vi "Variable_Local.vi"() -> ()   [LabVIEW 2016]
panel:
  out "String 2":string
  in  "String":string
  out "Waveform Chart":dbl(graph)
  in  "Stop Button":bool
  out "Numeric Control 2":i32
  out "Numeric Control":i32
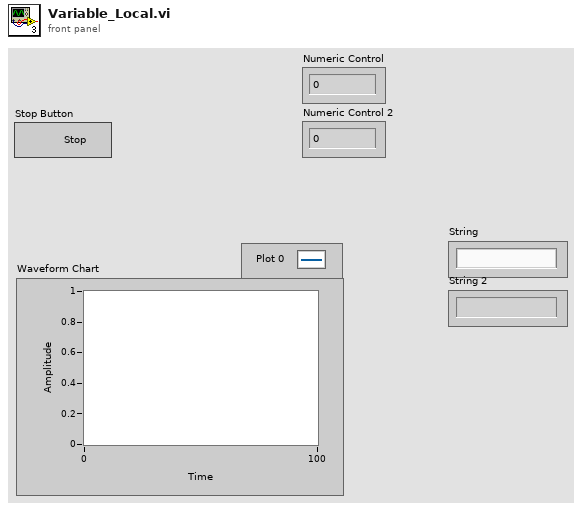
[diagram p1: front panel]
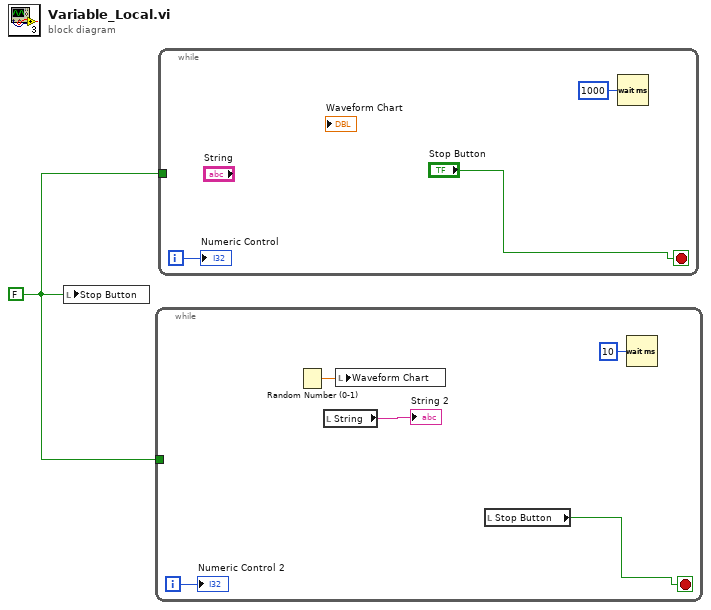
[diagram p0: block diagram]
diagram:
  w1 = FALSE ("Stop Button")
  n1 = local write "Stop Button"(w1) -> ()
  n2 = while {
    tunnel: w1 -> [_]
    i -> [w6]
    stop <- w4 stop-if-true
    n3 = Random Number (0-1)() -> (number: 0 to 1=w3:dbl)
    n4 = local read "String"() -> (→"String 2":string)
    n5 = local write "Waveform Chart"(w3) -> ()
    n6 = local read "Stop Button"() -> (w4:bool)
    n7 = Wait (ms)(milliseconds to wait=u32 10) -> ()  [unwired: 1 out]
    "Numeric Control 2" <- w6
  }
  n8 = while {
    tunnel: w1 -> [_]
    i -> [w9]
    stop <- "Stop Button" stop-if-true
    n9 = Wait (ms)(milliseconds to wait=u32 1000) -> ()  [unwired: 1 out]
    "Numeric Control" <- w9
  }
